vi "Light Enable.vi"(4 "Distance Refnum":refnum<vi>, 6 "Latitude Refnum":refnum<vi>, 7 "Enabled?":bool, 8 "error in (no error)":errorcluster, 9 "Longitude Refnum":refnum<vi>, 10 "Attenuation Refnum":refnum<vi>, 11 "Light color Refnum":refnum<vi>) -> (0 "error out":errorcluster)   [LabVIEW 2020, in "3D Plot.lvclass"]
uses:
  <vilib>/Math Plots/3D Math Plots/3D Plot/3D Plot/3D Plot.lvclass
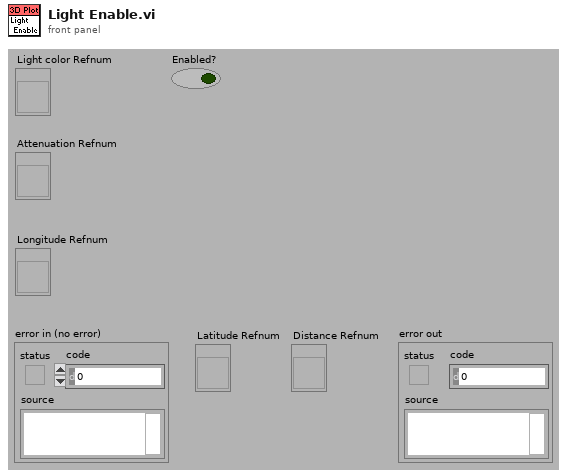
[diagram p1: front panel]
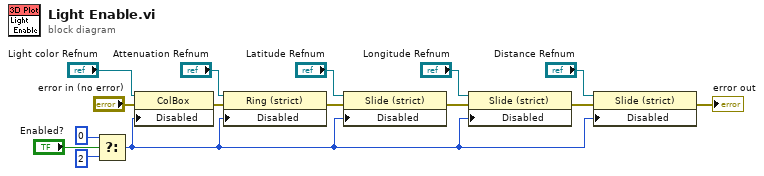
[diagram p0: block diagram]
diagram:
  n1 = Select(t=u8 0 ("Disabled"), s="Enabled?", f=u8 2) -> (s? t:f=w7:u8)
  n2 = property on="Property Node" class="ColBox"(reference="Light color Refnum", error in="error in (no error)", "Disabled"=w7) -> (error out=w6:errorcluster)  [unwired: 1 out]
  n3 = property on="Property Node" class="Ring (strict)"(reference="Attenuation Refnum", error in=w6, "Disabled"=w7) -> (error out=w5:errorcluster)  [unwired: 1 out]
  n4 = property on="Property Node" class="Slide (strict)"(reference="Latitude Refnum", error in=w5, "Disabled"=w7) -> (error out=w4:errorcluster)  [unwired: 1 out]
  n5 = property on="Property Node" class="Slide (strict)"(reference="Longitude Refnum", error in=w4, "Disabled"=w7) -> (error out=w3:errorcluster)  [unwired: 1 out]
  n6 = property on="Property Node" class="Slide (strict)"(reference="Distance Refnum", error in=w3, "Disabled"=w7) -> (error out=→"error out":errorcluster)  [unwired: 1 out]
